vi "FFT.vi"   [LabVIEW 2017, in "NI_AALPro.lvlib"]
doc: "Computes the fast Fourier transform (FFT) of the input sequence <B>X</B>. Wire data to the <B>X</B> input to determine the polymorphic instance to use or manually select the instance."
uses:
  <vilib>/Analysis/NI_AALPro.lvlib
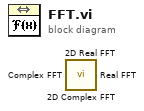
[diagram p0: block diagram]
diagram:
  n1 = call <vilib>:"2D Complex FFT.vi"() -> ()  [unwired: 10 in, 2 out]
  n2 = call <vilib>:"2D Real FFT.vi"() -> ()  [unwired: 10 in, 2 out]
  n3 = call <vilib>:"Complex FFT.vi"() -> ()  [unwired: 10 in, 2 out]
  n4 = call <vilib>:"Real FFT.vi"() -> ()  [unwired: 10 in, 2 out]
